vi "createPathToFile.vi"(10 "Pasta":string, 11 "Nome":string) -> (3 "path":path)   [LabVIEW 2013]
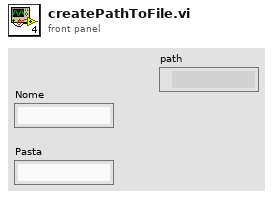
[diagram p1: front panel]
types:
  T1 = enum16{"open", "replace", "create", "open or create", "replace or create", "replace or create with confirmation"}
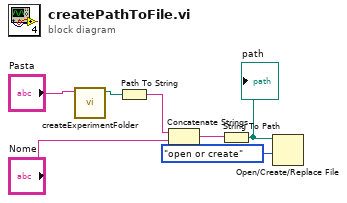
[diagram p0: block diagram]
diagram:
  n1 = call "createExperimentFolder.vi"("Experiment Name"="Pasta") -> ("created path"=w2:path)  [unwired: 10 in]
  n2 = Path To String(path=w2) -> (string=w3:string)
  n3 = Concatenate Strings(w3, "Nome") -> (w5:string)
  n4 = String To Path(string=w5) -> (path=w6:path)
  "path" <- w6
  n5 = Open/Create/Replace File(file path (use dialog)=w6, operation (0:open)=T1."open or create") -> ()  [unwired: 4 in, 3 out]
